vi "CenterSize to StartEnd or Rect-4C.vi"(4 "Resolution":u16=800, 6 "Size":dbl=2.0, 7 "Center":dbl) -> (0 "Rect-4C":cluster{"left":i16, "right":i16}={"left"=0, "right"=400}, 2 "End":dbl, 3 "Start":dbl=-1.0)   [LabVIEW 2018]
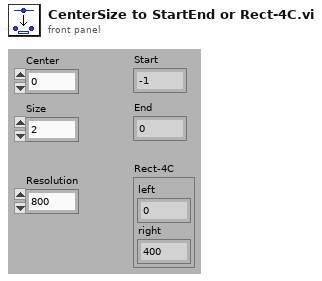
[diagram p1: front panel]
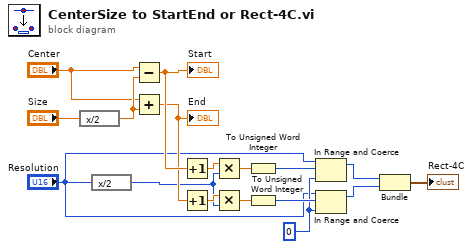
[diagram p0: block diagram]
diagram:
  w3 = u16 0 ("upper limit")
  n1 = expression code="x/2"("Size") -> (w16:dbl)
  n2 = expression code="x/2"("Resolution") -> (w10:u16)
  n3 = Subtract(x="Center", y=w16) -> (x-y=w13:dbl)
  "Start" <- w13
  n4 = Add(x="Center", y=w16) -> (x+y=w11:dbl)
  "End" <- w11
  n5 = Increment(x=w13) -> (x+1=w14:dbl)
  n6 = Increment(x=w11) -> (x+1=w12:dbl)
  n7 = Multiply(x=w14, y=w10) -> (x*y=w8:dbl)
  n8 = Multiply(x=w12, y=w10) -> (x*y=w6:dbl)
  n9 = To Unsigned Word Integer(number=w8) -> (unsigned 16bit integer=w7:u16)
  n10 = To Unsigned Word Integer(number=w6) -> (unsigned 16bit integer=w5:u16)
  n11 = In Range and Coerce(upper limit="Resolution", x=w7, lower limit=w3) -> (coerced(x)=w4:u16)  [unwired: 1 out]
  n12 = In Range and Coerce(upper limit="Resolution", x=w5, lower limit=w3) -> (coerced(x)=w1:u16)  [unwired: 1 out]
  n13 = Bundle("Resolution"=w4, "Resolution"=w1) -> (→"Rect-4C":cluster{"Resolution":u16, "Resolution":u16})  [unwired: 1 in]
